vi "Set Error Reporting.vi"(8 "error in (no error)":errorcluster, 10 "Error Reporting":T1, 11 "VisaComms in":refnum<class "VisaComms.lvclass">) -> (0 "error out":errorcluster, 3 "VisaComms out":refnum<class "VisaComms.lvclass">)   [LabVIEW 2020, in "CTI.lvlib" / "VisaComms.lvclass"]
uses:
  VisaComms.lvclass
  Error Reporting.ctl
  VisaComms.lvclass/VisaComms.ctl
  CTI.lvlib
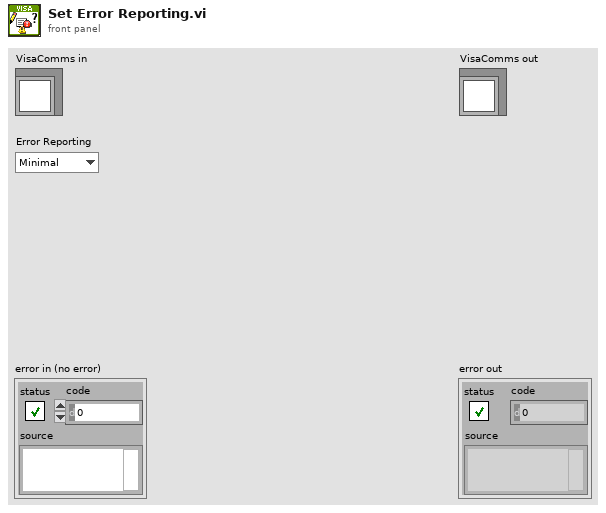
[diagram p1: front panel]
types:
  T1 = typedef "CTI.lvlib/Error Reporting.ctl" = enum16{"Minimal", "Moderate", "Full"}
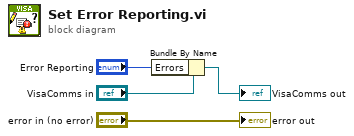
[diagram p0: block diagram]
diagram:
  n1 = Bundle By Name(cluster="VisaComms in", "Errors"="Error Reporting") -> (→"VisaComms out":refnum<class "VisaComms.lvclass">)
  "error out" <- "error in (no error)"
